vi "DATA_TRYL_VI.vi"() -> ()   [LabVIEW 2022 SP3]
uses:
  <extravilib>/ChannelInstances/Stream-a[.](dbl)/Read With Abort.vi
  <extravilib>/ChannelInstances/Stream-a[.](dbl)/EndpointRead.vi
  <extravilib>/ChannelInstances/Stream-a[.](dbl)/Instantiate.vi
  <extravilib>/ChannelInstances/Stream-a[.](dbl)/)Channel.vi
  <resource>/ChannelSupport/_ChannelSupport/WaitIfNeeded.vi
  <extravilib>/ChannelInstances/Stream-a[.](dbl).lvlib
panel:
  in  "stop":bool
  out "TrykLav":dbl[](array[numeric])
  out "TrykHoej":dbl[](array[numeric])
  out "Counter_Array":dbl[](array[numeric])
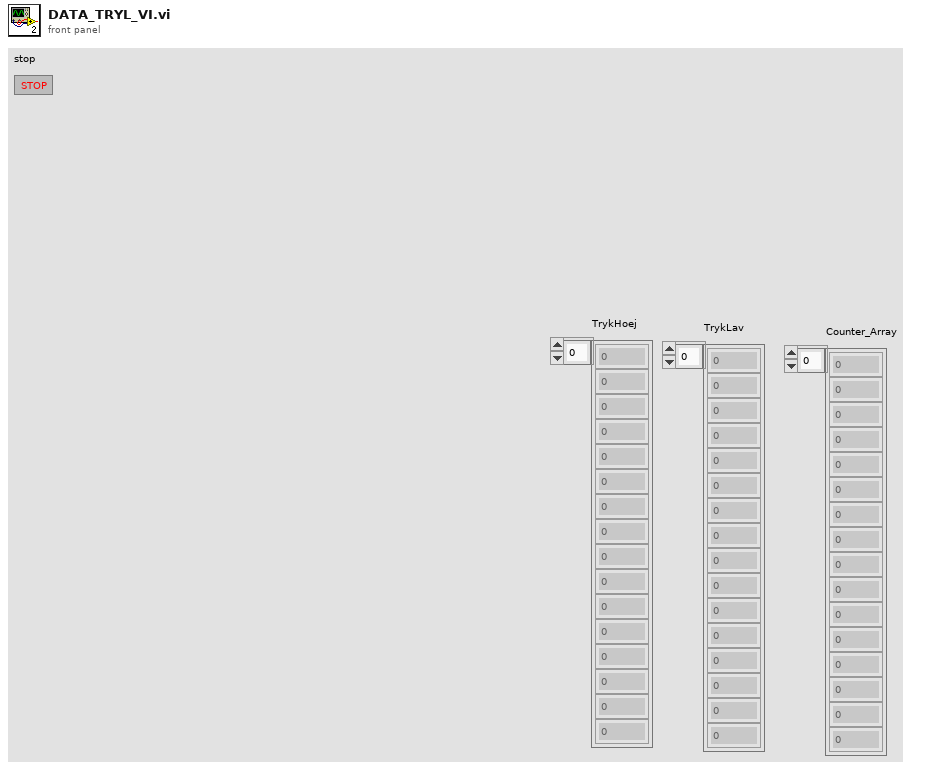
[diagram p1: front panel]
types:
  T1 = typedef "Stream-a[.](dbl).lvlib/)Channel.ctl" = refnum<queue>
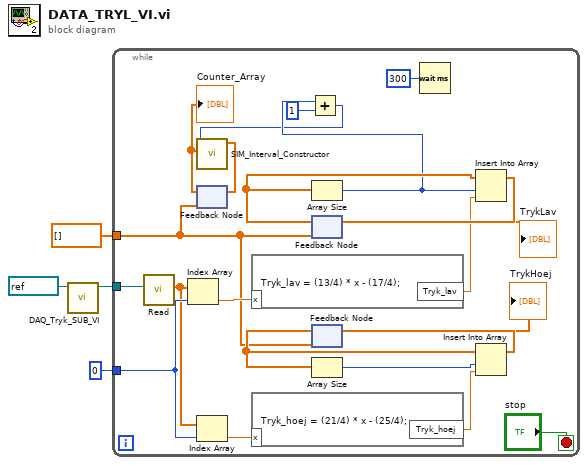
[diagram p0: block diagram]
diagram:
  n1 = call "DAQ_Tryk_SUB_VI.vi"("task in"=refnum<k21> "Tryk") -> ("channel"=w4:T1)  [unwired: 10 in]
  n2 = while {
    tunnel: w4 -> [w24]
    tunnel: 0 ("index") -> [w22]
    tunnel: dbl[] [] -> [w10]
    stop <- "stop" stop-if-true
    n3 = call <extravilib>:"Read.vi"("channel"=w24) -> ("element"=w21:dbl[])  [unwired: 6 in, 4 out]
    n4 = Index Array(array=w21, index=w22) -> (element=w20:dbl)
    n5 = feedback #1(w10) -> (w19:dbl[])
    "Counter_Array" <- w19
    n6 = Index Array(array=w21, index=w22) -> (element=w23:dbl)
    n7 = formula code="Tryk_lav = (13/4) * x - (17/4);"("x"=w20) -> ("Tryk_lav"=w15:dbl)
    n8 = formula code="Tryk_hoej = (21/4) * x - (25/4);"("x"=w23) -> ("Tryk_hoej"=w11:dbl)
    n9 = feedback #2(w10) -> (w16:dbl[])
    "TrykLav" <- w16
    n10 = Array Size(array=w16) -> (size(s)=w7:i32)
    n11 = Add(x=w7, y=1) -> (x+y=w5:i32)
    n12 = call "SIM_Interval_Constructor.vi"("History Data in"=w19, "size(s)"=w5) -> ("History Data out"=w18:dbl[])  [unwired: 9 in]
    n13 = feedback-in #1(w18) -> ()
    n14 = feedback #3(w10) -> (w13:dbl[])
    "TrykHoej" <- w13
    n15 = Array Size(array=w13) -> (size(s)=w12:i32)
    n16 = Wait (ms)(milliseconds to wait=u32 300) -> ()  [unwired: 1 out]
    n17 = Insert Into Array(array=w16, index=w7, new element=w15) -> (w17:dbl[])
    n18 = feedback-in #2(w17) -> ()
    n19 = Insert Into Array(array=w13, index=w12, new element=w11) -> (w14:dbl[])
    n20 = feedback-in #3(w14) -> ()
  }
